vi "To Waveform.vi"(8 "error in (no error)":errorcluster, 11 "Time Stamp in":refnum<class "Time Stamp.lvclass">) -> (0 "error out":errorcluster, 1 "Success?":bool, 3 "Waveform Array":waveform(dbl)[](array[waveform]))   [LabVIEW 2020, in "Data.lvlib" / "Time Stamp.lvclass"]
doc: "Interpret 'Data' as a Waveform Array. If impossible 'Success?' is set to FALSE"
uses:
  Time Stamp.lvclass
  Time Stamp.lvclass/Time Stamp.ctl
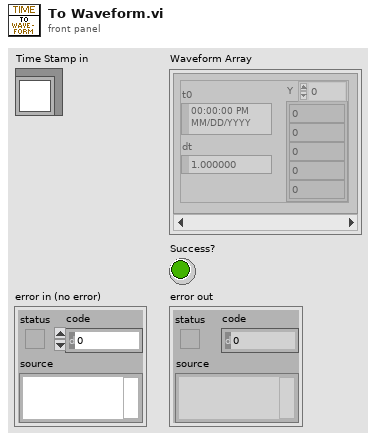
[diagram p1: front panel]
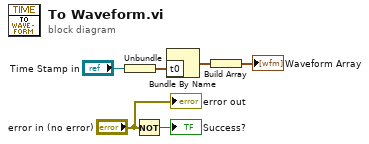
[diagram p0: block diagram]
diagram:
  n1 = Unbundle("Time Stamp in") -> (w6:timestamp)
  n2 = Not(x="error in (no error)") -> (.not. x?=→"Success?":bool)
  n3 = Bundle By Name("t0"=w6) -> (w4:waveform(dbl))  [unwired: 1 in]
  n4 = Build Array(w4) -> (→"Waveform Array":waveform(dbl)[])
  "error out" <- "error in (no error)"
